vi "Read Custom initialization.vi"(11 "Toggle 8 in":refnum<class "Toggle 8.lvclass">) -> (2 "Custom initialization":T1, 3 "Toggle 8 out":refnum<class "Toggle 8.lvclass">)   [LabVIEW 2020, in "Toggle 8.lvclass"]
uses:
  Toggle 8.lvclass
  Toggle 8.lvclass/Toggle 8.ctl
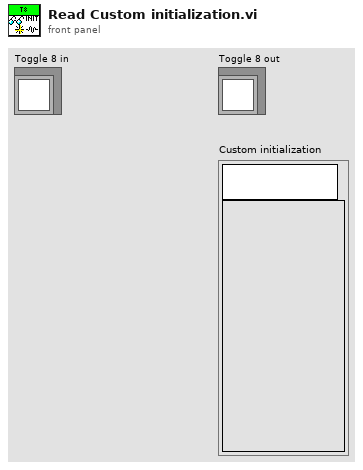
[diagram p1: front panel]
types:
  T1 = cluster{"Enable":bool, "User init values":string}
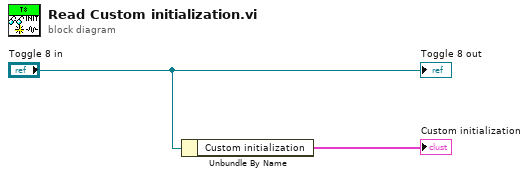
[diagram p0: block diagram]
diagram:
  n1 = Unbundle By Name("Toggle 8 in") -> ("Custom initialization"=→"Custom initialization":T1)
  "Toggle 8 out" <- "Toggle 8 in"
